vi "Read Resource Data ref.vi"(8 "error in (no error)":errorcluster, 11 "Menu Data in":refnum<class "Menu Data.lvclass">) -> (0 "error out":errorcluster, 2 "Resource Data ref":refnum<data-value>, 3 "Menu Data out":refnum<class "Menu Data.lvclass">)   [LabVIEW 2013, in "SET Project Data.lvlib" / "Menu Data.lvclass"]
uses:
  Menu Data.lvclass
  Resource Data Class/Resource Data.lvclass
  Menu Data.lvclass/Menu Data.ctl
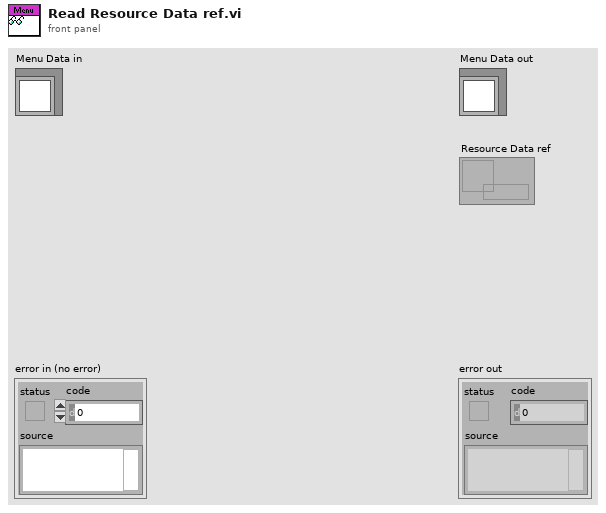
[diagram p1: front panel]
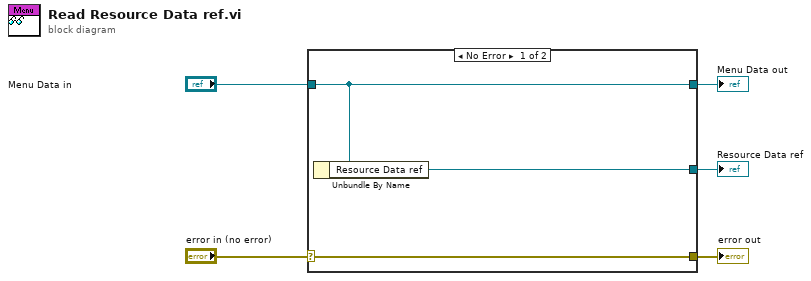
[diagram p0: block diagram]
diagram:
  n1 = case shown="No Error" "error in (no error)" {
    selector: "error in (no error)" -> [w8 w9]
    tunnel: [w8 w9] -> w4
    tunnel: [w7 w10] -> w2
    tunnel: "Menu Data in" -> [w7 w10]
    tunnel: [w6 _] -> w1
    frame No Error {
      n2 = Unbundle By Name(w7) -> ("Resource Data ref"=w6:refnum<data-value>)
    }
    frame Error {
    }
  }
  "error out" <- w4
  "Menu Data out" <- w2
  "Resource Data ref" <- w1
